vi "CameraCheckROI.vi"(8 "error in (no error)":errorcluster, 10 "ROI_in":T1, 11 "IMAQdx in":refnum<class "IMAQdx.lvclass">) -> (0 "error out":errorcluster, 2 "ROI_out":T1, 3 "IMAQdx out":refnum<class "IMAQdx.lvclass">)   [LabVIEW 2010, in "IMAQdx.lvclass"]
uses:
  <userlib>/BIAS2/classes/IMAQdx/IMAQdx.lvclass
  <userlib>/bias2/subvis/ROI_rect.ctl
  <userlib>/BIAS2/classes/IMAQdx/IMAQdx.lvclass/IMAQdx.ctl
  resource/objmgr/imaqdx.rc
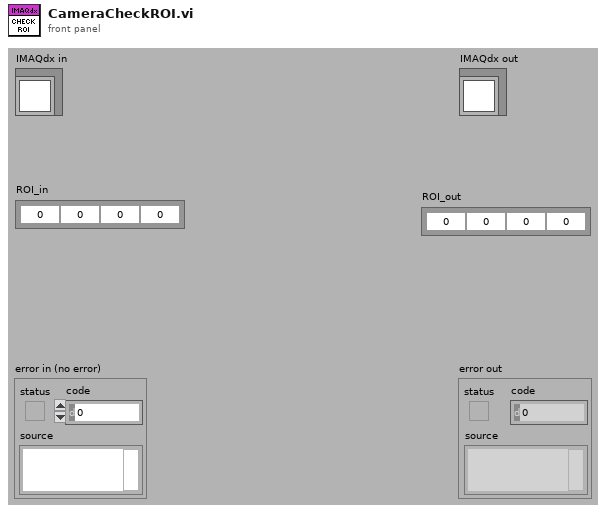
[diagram p1: front panel]
types:
  T1 = typedef "ROI_rect.ctl" = cluster{"left":i32, "top":i32, "right":i32, "bottom":i32}
  T2 = cluster{"ValueU32":u32, "ValueU32":u32, "ValueU32":u32, "ValueU32":u32}
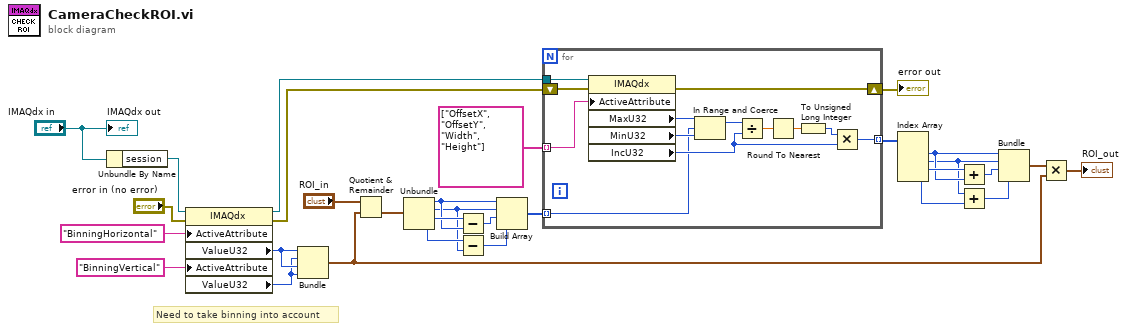
[diagram p0: block diagram]
diagram:
  # "Need to take binning into account"
  n1 = Unbundle By Name("IMAQdx in") -> ("session"=w3:refnum<k21>)
  n2 = property class="IMAQdx"(reference=w3, error in="error in (no error)", "ActiveAttribute"="BinningHorizontal", "ActiveAttribute"="BinningVertical") -> (reference out=w2:refnum<k21>, error out=w1:errorcluster, "ValueU32"=w11:u32, "ValueU32"=w10:u32)
  n3 = Bundle("ValueU32"=w11, "ValueU32"=w10, "ValueU32"=w11, "ValueU32"=w10) -> (w5:T2)  [unwired: 1 in]
  n4 = Quotient & Remainder(x="ROI_in", y=w5) -> (floor(x/y)=w8:cluster{u32, u32, u32, u32})  [unwired: 1 out]
  n5 = Unbundle(w8) -> (w28:u32, w27:u32, w30:u32, w29:u32)
  n6 = Subtract(x=w30, y=w28) -> (x-y=w26:u32)
  n7 = Subtract(x=w29, y=w27) -> (x-y=w25:u32)
  n8 = Build Array(w28, w27, w26, w25) -> (w24:u32[])
  n9 = for {
    tunnel: w24 -> [w31] mode=indexing
    tunnel: string[] ["OffsetX", "OffsetY", "Width", "Height"] -> [w41] mode=indexing
    shift-right: [w43] -> w21
    shift-left: w1 -> [w42]
    tunnel: w2 -> [w40]
    tunnel: [w32] -> w20 mode=indexing
    n10 = property class="IMAQdx"(reference=w40, error in=w42, "ActiveAttribute"=w41) -> (error out=w43:errorcluster, "MaxU32"=w37:u32, "MinU32"=w36:u32, "IncU32"=w33:u32)  [unwired: 1 out]
    n11 = In Range and Coerce(upper limit=w37, x=w31, lower limit=w36) -> (coerced(x)=w39:u32)  [unwired: 1 out]
    n12 = Divide(x=w39, y=w33) -> (x/y=w38:dbl)
    n13 = Round To Nearest(number=w38) -> (nearest integer value=w35:dbl)
    n14 = To Unsigned Long Integer(number=w35) -> (unsigned 32bit integer=w34:u32)
    n15 = Multiply(x=w34, y=w33) -> (x*y=w32:u32)
  }
  "error out" <- w21
  n16 = Index Array(array=w20) -> (element #1=w17:u32, element #2=w16:u32, element #3=w19:u32, element #4=w18:u32)  [unwired: 4 in]
  n17 = Add(x=w19, y=w17) -> (x+y=w15:u32)
  n18 = Add(x=w16, y=w18) -> (x+y=w14:u32)
  n19 = Bundle(w17, w16, w15, w14) -> (w7:cluster{u32, u32, u32, u32})  [unwired: 1 in]
  n20 = Multiply(x=w7, y=w5) -> (x*y=→"ROI_out":cluster{u32, u32, u32, u32})
  "IMAQdx out" <- "IMAQdx in"
